vi "X509_NAME_get_string.vi"(8 "error in (no error)":errorcluster, 10 "X509_Name":u64, 11 "X509-Cert in":refnum<class "X509-Cert.lvclass">) -> (0 "error out":errorcluster, 2 "X509 Name String":string, 3 "X509-Cert out":refnum<class "X509-Cert.lvclass">)   [LabVIEW 2013, in "SSL_Lib.lvlib" / "X509-Cert.lvclass"]
uses:
  X509-Cert.lvclass
  SSL-Lib/SSL-Lib.lvclass
  BIO/BIO.lvclass
panel:
  out "bytes written":i32
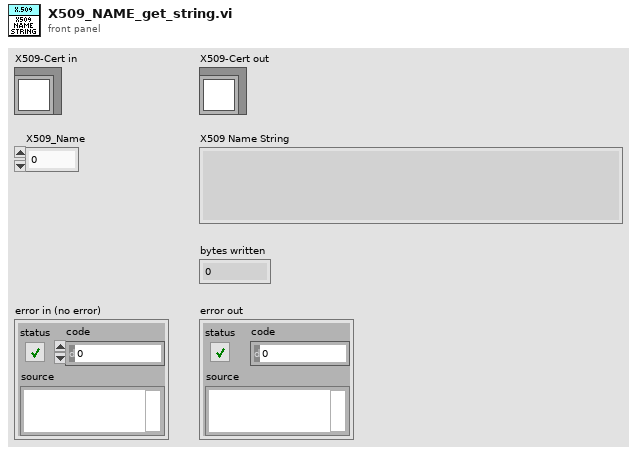
[diagram p1: front panel]
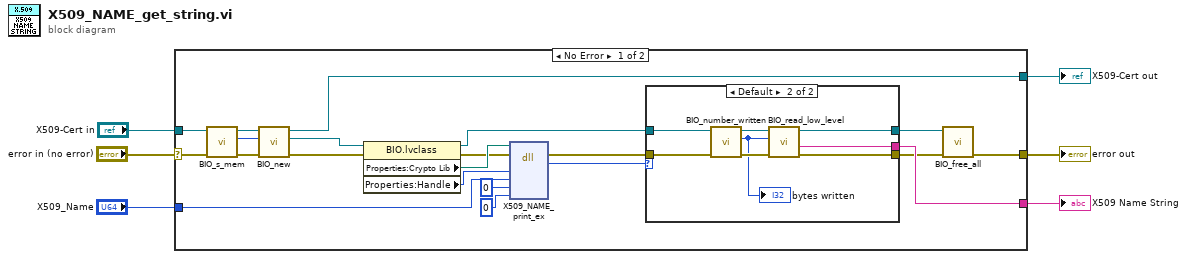
[diagram p0: block diagram]
diagram:
  n1 = case shown="No Error" "error in (no error)" {
    selector: "error in (no error)" -> [w10 w38]
    tunnel: "X509_Name" -> [w20 _]
    tunnel: [w16 _] -> w5
    tunnel: [w15 w38] -> w4
    tunnel: [w13 w39] -> w3
    tunnel: "X509-Cert in" -> [w12 w39]
    frame No Error {
      n2 = call "BIO_s_mem.vi"("error in (no error)"=w10, "SSL-Lib in"=w12) -> ("error out"=w7:errorcluster, "*BIO_Method"=w9:u64, "SSL-Lib out"=w8:refnum<class "X509-Cert.lvclass">)  [unwired: 7 in]
      n3 = call "BIO_new.vi"("error in (no error)"=w7, "*BIO_method"=w9, "SSL-Lib in"=w8) -> ("error out"=w17:errorcluster, "BIO out"=w24:refnum<class "BIO.lvclass">, "SSL-Lib out"=w13:refnum<class "X509-Cert.lvclass">)  [unwired: 6 in]
      n4 = property class="BIO.lvclass"(reference=w24, error in=w17) -> (reference out=w25:refnum<class "BIO.lvclass">, error out=w18:errorcluster, "Properties:Crypto Lib"=w27:path, "Properties:Handle"=w19:u64)
      n5 = dll-call lib="C:/Program Files (x86)/National Instruments/Shared/nissl/NIlibeay32.dll" fn="X509_NAME_print_ex"(path in=w27, error in=w18, "BIO"=w19, "X509_Name"=w20, "indent"=0, "flags"=u32 0) -> (error out=w23:errorcluster, "return type"=w26:i32)  [unwired: 5 in, 1 out]
      n6 = case shown="Default" w26 {
        tunnel: [w28 w35] -> w11
        tunnel: [w29 w33] -> w14
        tunnel: [_ w32] -> w16
        tunnel: w23 -> [w28 w31]
        tunnel: w25 -> [w29 w30]
        frame ..0 {
        }
        frame Default {
          n7 = call "BIO_number_written.vi"("error in (no error)"=w31, "BIO in"=w30) -> ("error out"=w37:errorcluster, "bytes written"=w36:i32, "BIO out"=w34:refnum<class "BIO.lvclass">)  [unwired: 7 in]
          "bytes written" <- w36
          n8 = call "BIO_read_low_level.vi"("error in (no error)"=w37, "bytes to read"=w36, "BIO in"=w34) -> ("error out"=w35:errorcluster, "buf"=w32:string, "BIO out"=w33:refnum<class "BIO.lvclass">)  [unwired: 5 in, 1 out]
        }
      }
      n9 = call "BIO_free_all.vi"("error in (no error)"=w11, "BIO in"=w14) -> ("error out"=w15:errorcluster)  [unwired: 9 in]
    }
    frame Error {
    }
  }
  "X509 Name String" <- w5
  "error out" <- w4
  "X509-Cert out" <- w3
